vi "Parser_SERVER.vi"(8 "error in (no error)":errorcluster, 10 "connection in":T1, 11 "Control in":refnum<class "Control-Server.lvclass">) -> (0 "error out":errorcluster, 2 "# clients":i32)   [LabVIEW 2015]
uses:
  Classes/Control/Control-Server/Control-Server.lvclass
  <vilib>/NI/STM/TCP/TCP Connection Info.ctl
  <vilib>/NI/STM/SubVIs/MetaDataElement.ctl
  <vilib>/NI/STM/Connection Manager/TCP/TCP Connection Method.ctl
  Clusters-def/OSc-Demand-Read.ctl
  Clusters-def/DL-Com-MoveAxis.ctl
  Clusters-def/Det-Read.ctl
  Clusters-def/Parameters_measurement_def.ctl
  <vilib>/NI/STM/TCP/Read Message (TCP).vi
  <vilib>/NI/STM/NI STM.lvlib
  Classes/Delay Line/DelayLine.lvclass
  Classes/Detector/Detector.lvclass
  Classes/Oscilloscope/Oscilloscope.lvclass
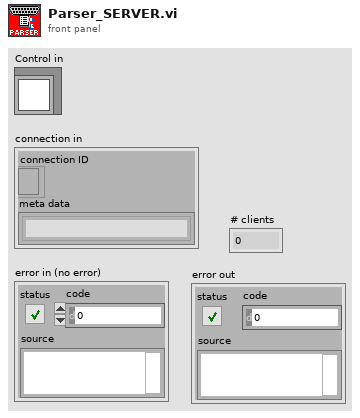
[diagram p1: front panel]
types:
  T1 = typedef "NI STM.lvlib/TCP Connection Info.ctl" = cluster{"connection ID":refnum<k5>, "meta data":T2[]}
  T2 = typedef "NI STM.lvlib/MetaDataElement.ctl" = string
  T3 = typedef "NI STM.lvlib/TCP Connection Method.ctl" = enum16{"Initialize", "Add Connection", "Set Properties", "Get Connection(s)", "Remove Connection", "Remove All Connections", "Get Connection Count"}
  T4 = typedef "NI STM.lvlib/TCP Connection Properties.ctl" = cluster{"Name":string, "Address":string, "Custom":string}
  T5 = typedef "Oscilloscope.lvclass/OSc-Demand-Read.ctl" = cluster{"ON/OFF":bool, "Channels":u16[]}
  T6 = typedef "DelayLine.lvclass/DL-Com-MoveAxis.ctl" = cluster{"Axis":i32, "Where":dbl, "How":u16}
  T7 = typedef "Detector.lvclass/Det-Read.ctl" = cluster{"# scans":i32, "All":bool, "Parameters of measurement":T8}
  T8 = typedef "Parameters_measurement_def.ctl" = cluster{"ODmin":dbl, "ODmax":dbl, "Aq contol":enum32{"fixed", "automatic", "fixed-auto"}, "Wavelength_fix_index":i32, "WCM_limits":cluster{"WCM_min":dbl, "WCM_max":dbl, "WCM_value":dbl}, "WCM_corrections":bool, "#cycles max":i32}
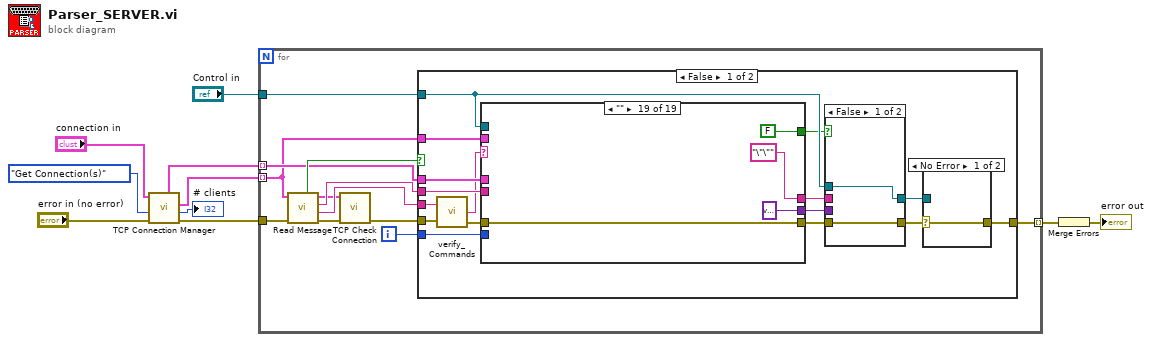
[diagram p0: block diagram]
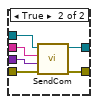
[diagram p2: hidden frame]
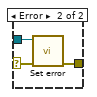
[diagram p3: hidden frame]
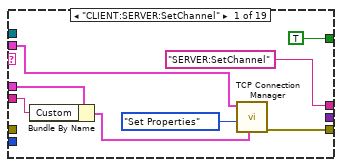
[diagram p4: hidden frame]
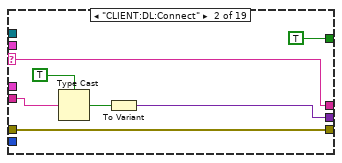
[diagram p5: hidden frame]
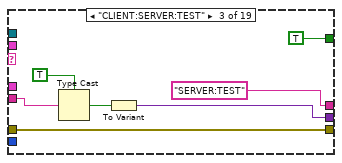
[diagram p6: hidden frame]
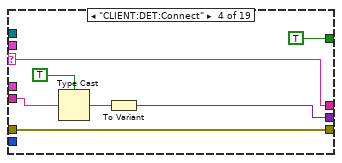
[diagram p7: hidden frame]
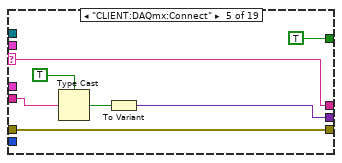
[diagram p8: hidden frame]
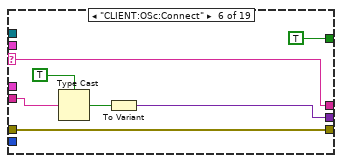
[diagram p9: hidden frame]
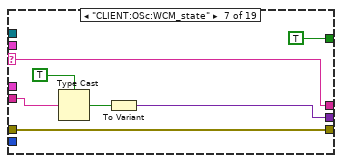
[diagram p10: hidden frame]
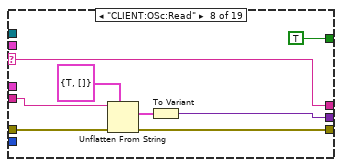
[diagram p11: hidden frame]
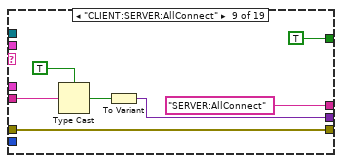
[diagram p12: hidden frame]
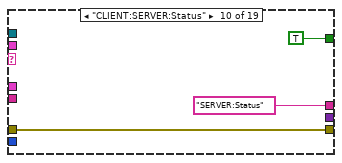
[diagram p13: hidden frame]
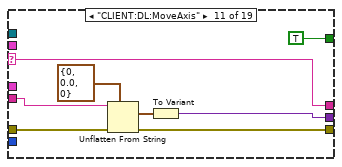
[diagram p14: hidden frame]
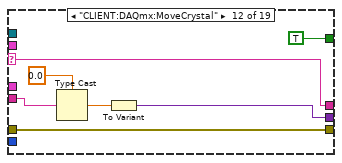
[diagram p15: hidden frame]
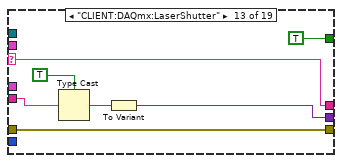
[diagram p16: hidden frame]
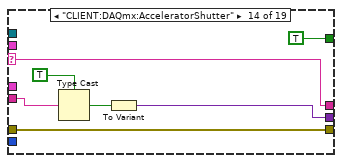
[diagram p17: hidden frame]
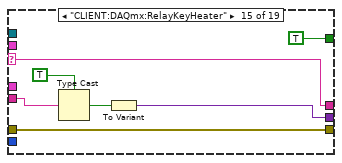
[diagram p18: hidden frame]
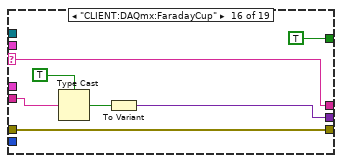
[diagram p19: hidden frame]
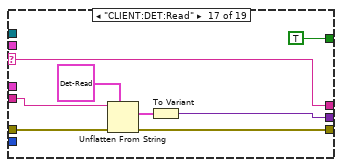
[diagram p20: hidden frame]
diagram:
  n1 = call <vilib>:"TCP Connection Manager.vi"("error in"="error in (no error)", "method"=TCP_Connection_Method."Get Connection(s)", "connection in"="connection in") -> ("error out"=w3:errorcluster, "number of connections"=→"# clients":i32, "all connections"=w6:T1[], "all properties"=w5:T4[])  [unwired: 3 in, 2 out]
  n2 = for {
    tunnel: w6 -> [w16] mode=indexing
    tunnel: w5 -> [w17] mode=indexing
    tunnel: w3 -> [w14]
    tunnel: "Control in" -> [w13]
    tunnel: [w11] -> w2 mode=indexing
    i -> [w18]
    n3 = call-poly <vilib>:"Read Message.vi"("error in"=w14, "connection info in"=w16) -> ("error out"=w19:errorcluster, "name"=w22:T2, "data string"=w21:string, "connection info out"=w15:T1, "timed out?"=w20:bool)  [unwired: 4 in, 1 out]
    n4 = call <vilib>:"TCP Check Connection.vi"("error in"=w19, "connection in"=w15) -> ("error out"=w12:errorcluster)  [unwired: 7 in, 2 out]
    n5 = case shown="False" w20 {
      tunnel: w22 -> [w28 _]
      tunnel: w21 -> [w35 _]
      tunnel: w16 -> [w38 _]
      tunnel: w18 -> [w37 _]
      tunnel: w17 -> [w36 _]
      tunnel: w13 -> [w30 _]
      tunnel: w12 -> [w27 w178]
      tunnel: [w31 w178] -> w11
      frame False {
        n6 = call "verify_Commands.vi"("Command"=w28, "error in"=w27) -> ("Command out"=w29:string, "error out"=w26:errorcluster)  [unwired: 1 out]
        n7 = case shown="\"\"" w29 {
          selector: w29 -> [_ w62 _ w79 w86 w93 w100 w108 _ _ w126 w132 w139 w146 w153 w160 w169 _ _]
          tunnel: w38 -> [w56 _ _ _ _ _ _ _ _ _ _ _ _ _ _ _ _ _ _]
          tunnel: w37 -> [_ _ _ _ _ _ _ _ _ _ _ _ _ _ _ _ _ _ _]
          tunnel: w36 -> [w58 _ _ _ _ _ _ _ _ _ _ _ _ _ _ _ _ _ _]
          tunnel: [w54 w63 w70 w76 w83 w90 w97 w101 w113 w118 w121 w128 w136 w143 w150 w157 w164 w173 w177] -> w33
          tunnel: w35 -> [w53 w64 w71 w77 w84 w91 w98 w104 w114 _ w123 w133 w140 w147 w154 w161 w166 _ _]
          tunnel: w30 -> [_ _ _ _ _ _ _ _ _ _ _ _ _ _ _ _ _ _ _]
          tunnel: w26 -> [_ w63 w70 w76 w83 w90 w97 w103 w113 w118 w122 w128 w136 w143 w150 w157 w165 w173 w177]
          tunnel: ["SERVER:SetChannel" w62 "SERVER:TEST" w79 w86 w93 w100 w108 "SERVER:AllConnect" "SERVER:Status" w126 w132 w139 w146 w153 w160 w169 "Unknown Command send to Parser" "\"\""] -> w34
          tunnel: [_ w60 w68 w74 w81 w88 w95 w107 w111 _ w125 w130 w137 w144 w151 w158 w168 variant ("Variant") variant ("Variant")] -> w32
          tunnel: [TRUE TRUE TRUE TRUE TRUE TRUE TRUE TRUE TRUE TRUE TRUE TRUE TRUE TRUE TRUE TRUE TRUE TRUE FALSE] -> w23
          frame "CLIENT:SERVER:SetChannel" {
            n8 = Bundle By Name(cluster=w58, "Custom"=w53) -> (w57:T4)
            n9 = call <vilib>:"TCP Connection Manager.vi"("properties in"=w57, "method"=TCP_Connection_Method."Set Properties", "connection in"=w56) -> ("error out"=w54:errorcluster)  [unwired: 3 in, 5 out]
          }
          frame "CLIENT:DL:Connect" {
            n10 = Type Cast(type=TRUE, x=w64) -> (*(type *) &x=w61:bool)
            n11 = To Variant(anything=w61) -> (Variant=w60:variant)
          }
          frame "CLIENT:SERVER:TEST" {
            n12 = Type Cast(type=TRUE, x=w71) -> (*(type *) &x=w69:bool)
            n13 = To Variant(anything=w69) -> (Variant=w68:variant)
          }
          frame "CLIENT:DET:Connect" {
            n14 = Type Cast(type=TRUE, x=w77) -> (*(type *) &x=w75:bool)
            n15 = To Variant(anything=w75) -> (Variant=w74:variant)
          }
          frame "CLIENT:DAQmx:Connect" {
            n16 = Type Cast(type=TRUE, x=w84) -> (*(type *) &x=w82:bool)
            n17 = To Variant(anything=w82) -> (Variant=w81:variant)
          }
          frame "CLIENT:OSc:Connect" {
            n18 = Type Cast(type=TRUE, x=w91) -> (*(type *) &x=w89:bool)
            n19 = To Variant(anything=w89) -> (Variant=w88:variant)
          }
          frame "CLIENT:OSc:WCM_state" {
            n20 = Type Cast(type=TRUE, x=w98) -> (*(type *) &x=w96:bool)
            n21 = To Variant(anything=w96) -> (Variant=w95:variant)
          }
          frame "CLIENT:OSc:Read" {
            n22 = Unflatten From String(type=T5 {"ON/OFF"=TRUE, "Channels"=[]}, binary string=w104, error in (no error)=w103) -> (value=w102:T5, error out=w101:errorcluster)  [unwired: 2 in, 1 out]
            n23 = To Variant(anything=w102) -> (Variant=w107:variant)
          }
          frame "CLIENT:SERVER:AllConnect" {
            n24 = Type Cast(type=TRUE, x=w114) -> (*(type *) &x=w112:bool)
            n25 = To Variant(anything=w112) -> (Variant=w111:variant)
          }
          frame "CLIENT:SERVER:Status" {
          }
          frame "CLIENT:DL:MoveAxis" {
            n26 = Unflatten From String(type=T6 {"Axis"=0, "Where"=0.0, "How"=0} ("output cluster"), binary string=w123, error in (no error)=w122) -> (value=w119:T6, error out=w121:errorcluster)  [unwired: 2 in, 1 out]
            n27 = To Variant(anything=w119) -> (Variant=w125:variant)
          }
          frame "CLIENT:DAQmx:MoveCrystal" {
            n28 = Type Cast(type=0.0, x=w133) -> (*(type *) &x=w131:dbl)
            n29 = To Variant(anything=w131) -> (Variant=w130:variant)
          }
          frame "CLIENT:DAQmx:LaserShutter" {
            n30 = Type Cast(type=TRUE, x=w140) -> (*(type *) &x=w138:bool)
            n31 = To Variant(anything=w138) -> (Variant=w137:variant)
          }
          frame "CLIENT:DAQmx:AcceleratorShutter" {
            n32 = Type Cast(type=TRUE, x=w147) -> (*(type *) &x=w145:bool)
            n33 = To Variant(anything=w145) -> (Variant=w144:variant)
          }
          frame "CLIENT:DAQmx:RelayKeyHeater" {
            n34 = Type Cast(type=TRUE, x=w154) -> (*(type *) &x=w152:bool)
            n35 = To Variant(anything=w152) -> (Variant=w151:variant)
          }
          frame "CLIENT:DAQmx:FaradayCup" {
            n36 = Type Cast(type=TRUE, x=w161) -> (*(type *) &x=w159:bool)
            n37 = To Variant(anything=w159) -> (Variant=w158:variant)
          }
          frame "CLIENT:DET:Read" {
            n38 = Unflatten From String(type=T7 {"# scans"=0, "All"=FALSE, "Parameters of measurement"={"ODmin"=0.0, "ODmax"=0.0, "Aq contol"=enum."fixed", "Wavelength_fix_index"=640, "WCM_limits"={"WCM_min"=0.0, "WCM_max"=0.0, "WCM_value"=0.0}, "WCM_corrections"=FALSE, "#cycles max"=5}} ("cluster"), binary string=w166, error in (no error)=w165) -> (value=w163:T7, error out=w164:errorcluster)  [unwired: 2 in, 1 out]
            n39 = To Variant(anything=w163) -> (Variant=w168:variant)
          }
          frame "Error", Default {
          }
          frame "" {
          }
        }
        n40 = case shown="False" w23 {
          tunnel: w34 -> [_ w46]
          tunnel: w33 -> [w39 w45]
          tunnel: w32 -> [_ w44]
          tunnel: w30 -> [w40 w43]
          tunnel: [w40 w42] -> w25
          tunnel: [w39 w41] -> w24
          frame False {
          }
          frame True {
            n41 = call "SendCom.vi"("error in (no error)"=w45, "data"=w44, "Commands"=w46, "Control in"=w43) -> ("error out"=w41:errorcluster, "Control out"=w42:refnum<class "Control-Server.lvclass">)  [unwired: 6 in]
          }
        }
        n42 = case shown="No Error" w24 {
          selector: w24 -> [w47 w48]
          tunnel: [w47 w50] -> w31
          tunnel: w25 -> [_ w49]
          frame No Error {
          }
          frame Error {
            n43 = call "Set error.vi"("error in (no error)"=w48, "Control-Server in"=w49) -> ("error out"=w50:errorcluster)  [unwired: 8 in, 1 out]
          }
        }
      }
      frame True {
      }
    }
  }
  n44 = Merge Errors(w2) -> (→"error out":errorcluster)
